vi "SI656.vi"(0 "SI656 in":refnum<class "SI656.lvclass">, 1 "Limitation":bool=TRUE, 2 "From Turbine":T1, 3 "In1":dbl, 4 "In2":dbl, 5 "error in (no error)":errorcluster) -> (14 "SI656 out":refnum<class "SI656.lvclass">, 16 "PG Factor":dbl, 17 "PG 2nd Min in %":dbl, 19 "error out":errorcluster)   [LabVIEW 2022 SP3, in "SI656.lvclass"]
uses:
  SI656.lvclass
  SI656.lvclass/SI656.ctl
panel:
  # "SI656"
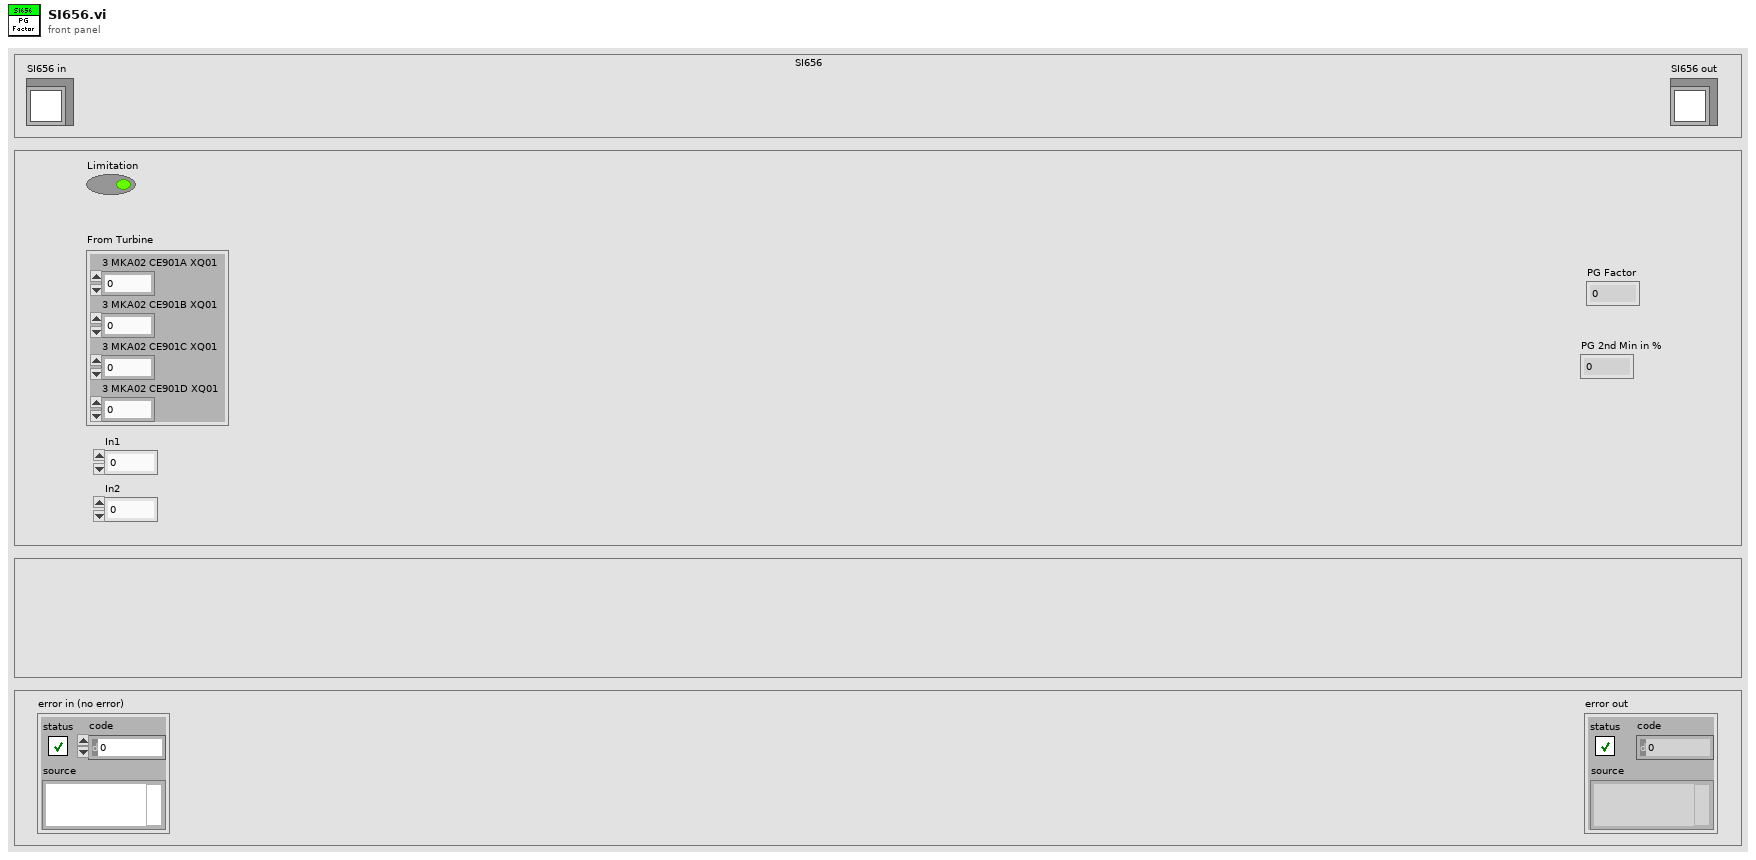
[diagram p1: front panel]
types:
  T1 = cluster{"3 MKA02 CE901A XQ01":dbl, "3 MKA02 CE901B XQ01":dbl, "3 MKA02 CE901C XQ01":dbl, "3 MKA02 CE901D XQ01":dbl}
  T2 = cluster{"LL":dbl, "OutLimMin":dbl, "OutLimMax":dbl, "UL":dbl, "In1":dbl, "In2":dbl, "Out1":dbl, "Out2":dbl, "Limitation":bool}
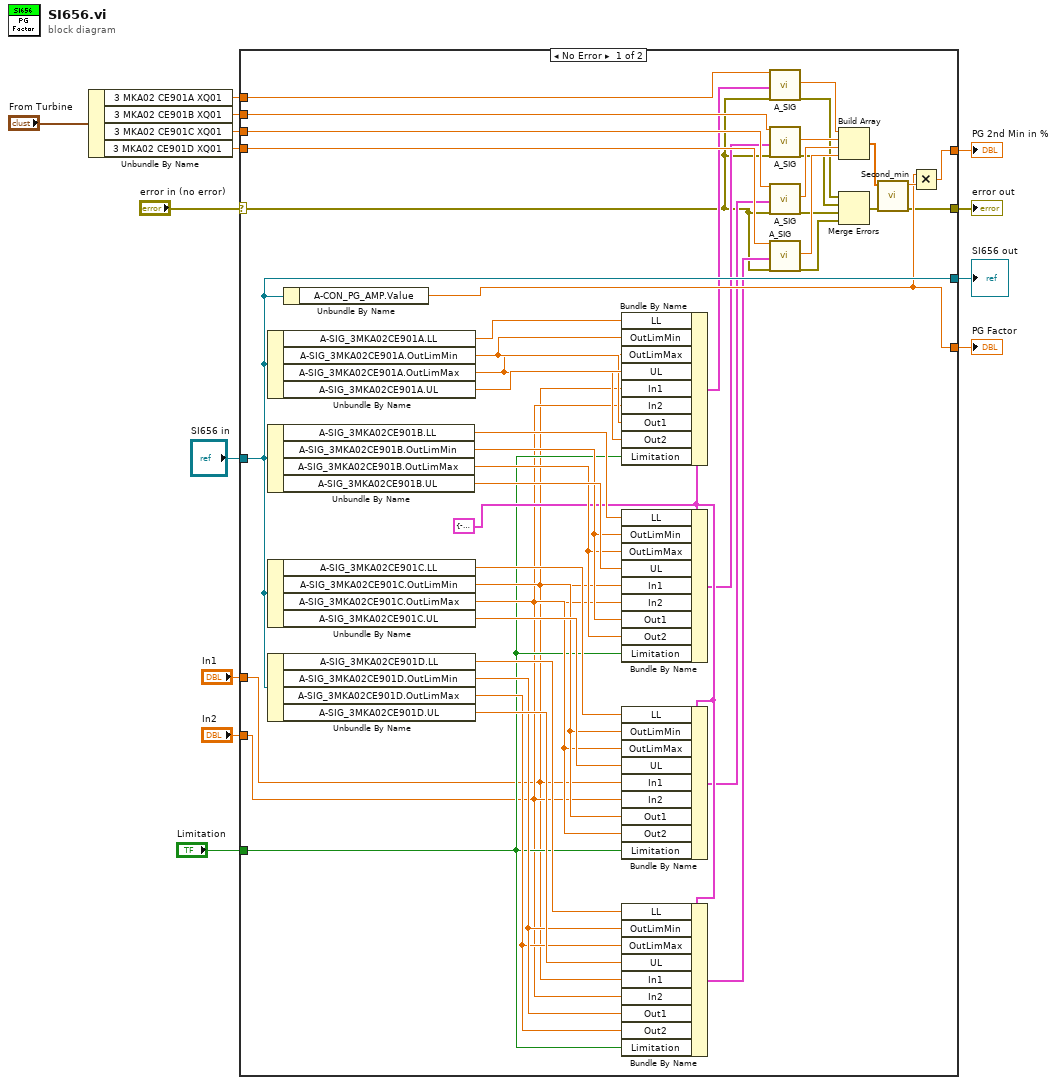
[diagram p0: block diagram]
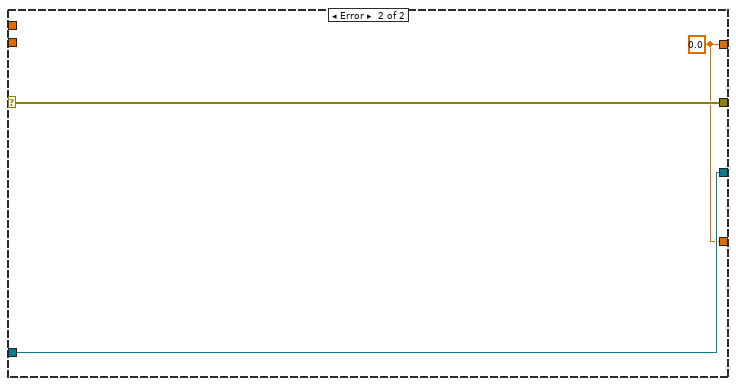
[diagram p2: hidden frame]
diagram:
  n1 = Unbundle By Name("From Turbine") -> ("3 MKA02 CE901A XQ01"=w8:dbl, "3 MKA02 CE901B XQ01"=w7:dbl, "3 MKA02 CE901C XQ01"=w6:dbl, "3 MKA02 CE901D XQ01"=w5:dbl)
  n2 = case shown="No Error" "error in (no error)" {
    selector: "error in (no error)" -> [w23 w61]
    tunnel: [w49 w61] -> w13
    tunnel: [w51 w60] -> w11
    tunnel: "SI656 in" -> [w51 w60]
    tunnel: w5 -> [w45 _]
    tunnel: w6 -> [w46 _]
    tunnel: w7 -> [w47 _]
    tunnel: w8 -> [w48 _]
    tunnel: [w52 w59] -> w10
    tunnel: [w50 w59] -> w4
    tunnel: "Limitation" -> [w17 _]
    tunnel: "In2" -> [w16 _]
    tunnel: "In1" -> [w15 _]
    frame No Error {
      w31 = T2 {"LL"=-47.0, "OutLimMin"=0.0, "OutLimMax"=1500.0, "UL"=1500.0, "In1"=4.0, "In2"=20.0, "Out1"=0.0, "Out2"=1500.0, "Limitation"=TRUE} ("Cluster")
      n3 = Unbundle By Name(w51) -> ("A-SIG_3MKA02CE901A.LL"=w44:dbl, "A-SIG_3MKA02CE901A.OutLimMin"=w42:dbl, "A-SIG_3MKA02CE901A.OutLimMax"=w41:dbl, "A-SIG_3MKA02CE901A.UL"=w43:dbl)
      n4 = Unbundle By Name(w51) -> ("A-SIG_3MKA02CE901B.LL"=w39:dbl, "A-SIG_3MKA02CE901B.OutLimMin"=w37:dbl, "A-SIG_3MKA02CE901B.OutLimMax"=w36:dbl, "A-SIG_3MKA02CE901B.UL"=w38:dbl)
      n5 = Unbundle By Name(w51) -> ("A-SIG_3MKA02CE901C.LL"=w35:dbl, "A-SIG_3MKA02CE901C.OutLimMin"=w33:dbl, "A-SIG_3MKA02CE901C.OutLimMax"=w32:dbl, "A-SIG_3MKA02CE901C.UL"=w34:dbl)
      n6 = Unbundle By Name(w51) -> ("A-SIG_3MKA02CE901D.LL"=w30:dbl, "A-SIG_3MKA02CE901D.OutLimMin"=w28:dbl, "A-SIG_3MKA02CE901D.OutLimMax"=w27:dbl, "A-SIG_3MKA02CE901D.UL"=w29:dbl)
      n7 = Unbundle By Name(w51) -> ("A-CON_PG_AMP.Value"=w50:dbl)
      n8 = Bundle By Name(cluster=w31, "LL"=w44, "OutLimMin"=w42, "OutLimMax"=w41, "UL"=w43, "In1"=w15, "In2"=w16, "Out1"=w42, "Out2"=w41, "Limitation"=w17) -> (w40:T2)
      n9 = Bundle By Name(cluster=w31, "LL"=w39, "OutLimMin"=w37, "OutLimMax"=w36, "UL"=w38, "In1"=w15, "In2"=w16, "Out1"=w37, "Out2"=w36, "Limitation"=w17) -> (w26:T2)
      n10 = Bundle By Name(cluster=w31, "LL"=w35, "OutLimMin"=w33, "OutLimMax"=w32, "UL"=w34, "In1"=w15, "In2"=w16, "Out1"=w33, "Out2"=w32, "Limitation"=w17) -> (w25:T2)
      n11 = Bundle By Name(cluster=w31, "LL"=w30, "OutLimMin"=w28, "OutLimMax"=w27, "UL"=w29, "In1"=w15, "In2"=w16, "Out1"=w28, "Out2"=w27, "Limitation"=w17) -> (w24:T2)
      n12 = call "A_SIG.vi"("Input(AI1)"=w48, "Cluster"=w40, "error in (no error)"=w23) -> ("AO1"=w58:dbl, "error out"=w22:errorcluster)  [unwired: 13 in, 2 out]
      n13 = call "A_SIG.vi"("Input(AI1)"=w47, "Cluster"=w26, "error in (no error)"=w23) -> ("AO1"=w57:dbl, "error out"=w21:errorcluster)  [unwired: 13 in, 2 out]
      n14 = call "A_SIG.vi"("Input(AI1)"=w46, "Cluster"=w25, "error in (no error)"=w23) -> ("AO1"=w56:dbl, "error out"=w20:errorcluster)  [unwired: 13 in, 2 out]
      n15 = call "A_SIG.vi"("Input(AI1)"=w45, "Cluster"=w24, "error in (no error)"=w23) -> ("AO1"=w55:dbl, "error out"=w19:errorcluster)  [unwired: 13 in, 2 out]
      n16 = Build Array(w58, w57, w56, w55) -> (w54:dbl[])
      n17 = Merge Errors(w22, w21, w20, w19) -> (w18:errorcluster)
      n18 = call "Second_min.vi"("error in (no error)"=w18, "Array"=w54) -> ("error IO"=w49:errorcluster, "output"=w53:dbl)  [unwired: 8 in]
      n19 = Multiply(x=w50, y=w53) -> (x*y=w52:dbl)
    }
    frame Error {
      w59 = 0.0
    }
  }
  "error out" <- w13
  "SI656 out" <- w11
  "PG Factor" <- w4
  "PG 2nd Min in %" <- w10
